vi "Sub_Calculate2DTemperatureSpread.vi"() -> ()   [LabVIEW 2018]
panel:
  out "Array":dbl[][](array[numeric])
  out "initialized array":dbl[][](array[numeric])
  in  "Sensor information":T1(array[cluster])
  in  "Simulation parameters":cluster{"Object height":u8, "Object width":u8}
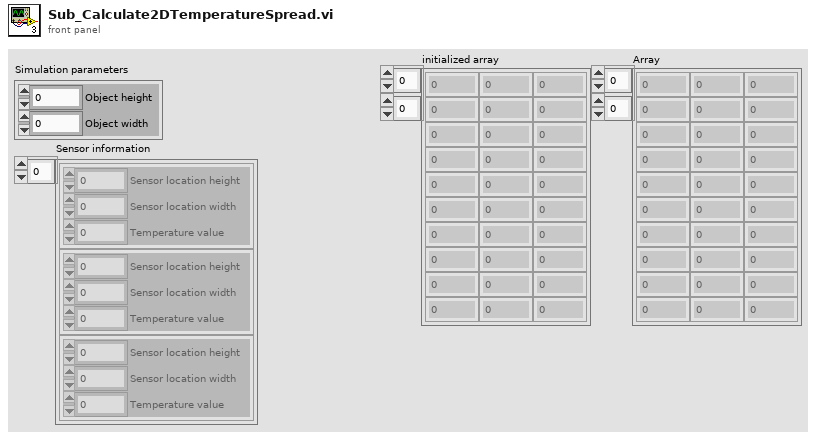
[diagram p1: front panel]
types:
  T1 = cluster{"Sensor location height":u8, "Sensor location width":u8, "Temperature value":dbl}[]
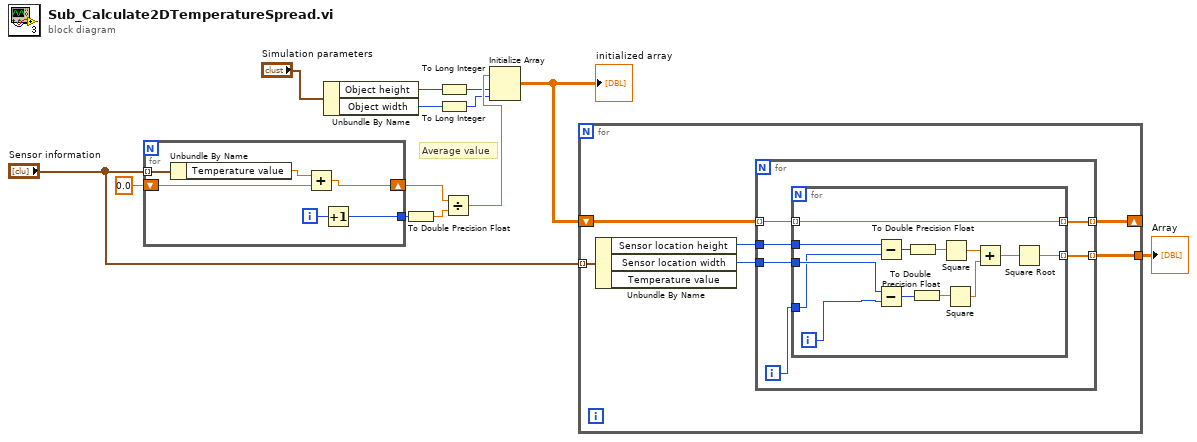
[diagram p0: block diagram]
diagram:
  # "Average value"
  n1 = for {
    tunnel: "Sensor information" -> [w19] mode=indexing
    shift-right: [w15] -> w9
    shift-left: 0.0 -> [w17]
    tunnel: [w14] -> w10
    i -> [w16]
    n2 = Unbundle By Name(w19) -> ("Temperature value"=w18:dbl)
    n3 = Add(x=w18, y=w17) -> (x+y=w15:dbl)
    n4 = Increment(x=w16) -> (x+1=w14:i32)
  }
  n5 = Unbundle By Name("Simulation parameters") -> ("Object height"=w4:u8, "Object width"=w12:u8)
  n6 = To Double Precision Float(number=w10) -> (double precision float=w5:dbl)
  n7 = To Long Integer(number=w4) -> (32bit integer=w3:i32)
  n8 = To Long Integer(number=w12) -> (32bit integer=w2:i32)
  n9 = Divide(x=w9, y=w5) -> (x/y=w8:dbl)
  n10 = Initialize Array(w8, w3, w2) -> (w6:dbl[][])
  "initialized array" <- w6
  n11 = for {
    tunnel: "Sensor information" -> [w24] mode=indexing
    shift-right: [w20] -> _
    shift-left: w6 -> [w25]
    tunnel: [w21] -> w1
    n12 = Unbundle By Name(w24) -> ("Sensor location height"=w23:u8, "Sensor location width"=w22:u8)  [unwired: 1 out]
    n13 = for {
      tunnel: w25 -> [w31] mode=indexing
      tunnel: w23 -> [w29]
      tunnel: w22 -> [w28]
      tunnel: [w27] -> w21 mode=indexing
      tunnel: [w26] -> w20 mode=indexing
      i -> [w30]
      n14 = for {
        tunnel: w31 -> [w35] mode=indexing
        tunnel: w30 -> [w33]
        tunnel: w29 -> [w44]
        tunnel: w28 -> [w39]
        tunnel: [w32] -> w27 mode=indexing
        tunnel: [w35] -> w26 mode=indexing
        i -> [w34]
        n15 = Subtract(x=w44, y=w33) -> (x-y=w43:i32)
        n16 = Subtract(x=w39, y=w34) -> (x-y=w40:i32)
        n17 = To Double Precision Float(number=w43) -> (double precision float=w42:dbl)
        n18 = To Double Precision Float(number=w40) -> (double precision float=w41:dbl)
        n19 = Square(x=w42) -> (x^2=w37:dbl)
        n20 = Square(x=w41) -> (x^2=w38:dbl)
        n21 = Add(x=w37, y=w38) -> (x+y=w36:dbl)
        n22 = Square Root(x=w36) -> (sqrt(x)=w32:dbl)
      }
    }
  }
  "Array" <- w1
